vi "create_full_endpoint.vi"(8 "error in (no error)":errorcluster, 11 "llm_openai_chatmodels in":refnum<class "llm_ollama_chatmodels.lvclass">) -> (0 "error out":errorcluster, 2 "endpoint":string, 3 "llm_openai_chatmodels out":refnum<class "llm_ollama_chatmodels.lvclass">)   [LabVIEW 2020, in "llm_ollama_chatmodels.lvclass"]
uses:
  llm_ollama_chatmodels.lvclass
  llm_ollama_chatmodels.lvclass/llm_ollama_chatmodels.ctl
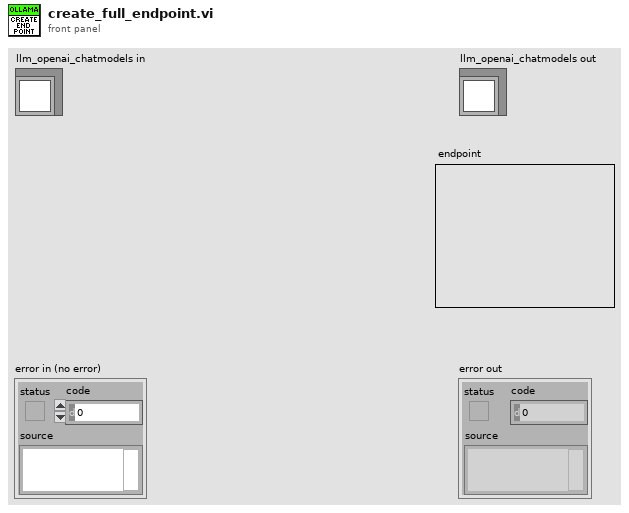
[diagram p1: front panel]
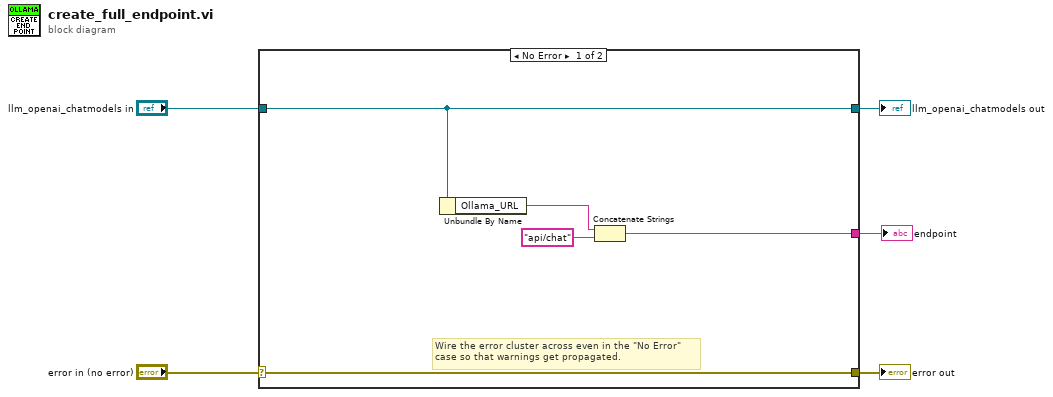
[diagram p0: block diagram]
diagram:
  n1 = case shown="No Error" "error in (no error)" {
    selector: "error in (no error)" -> [w10 w12]
    tunnel: [w10 w12] -> w4
    tunnel: [w8 w11] -> w2
    tunnel: "llm_openai_chatmodels in" -> [w8 w11]
    tunnel: [w6 _] -> w1
    frame No Error {
      # "Wire the error cluster across even in the \"No Error\"\ncase so that warnings get propagated."
      n2 = Unbundle By Name(w8) -> ("Ollama_URL"=w7:string)
      n3 = Concatenate Strings(w7, "api/chat" ("url")) -> (w6:string)
    }
    frame Error {
    }
  }
  "error out" <- w4
  "llm_openai_chatmodels out" <- w2
  "endpoint" <- w1
